vi "calculateWaveformTime.vi"(8 "error in (no error)":errorcluster, 11 "ChirpWave in":refnum<class "ChirpWave.lvclass">) -> (0 "error out":errorcluster, 2 "Waveform Time":dbl[unit], 3 "ChirpWave out":refnum<class "ChirpWave.lvclass">)   [LabVIEW 2015, in "ChirpWave.lvclass"]
uses:
  ChirpWave.lvclass
  ChirpWave.lvclass/ChirpWave.ctl
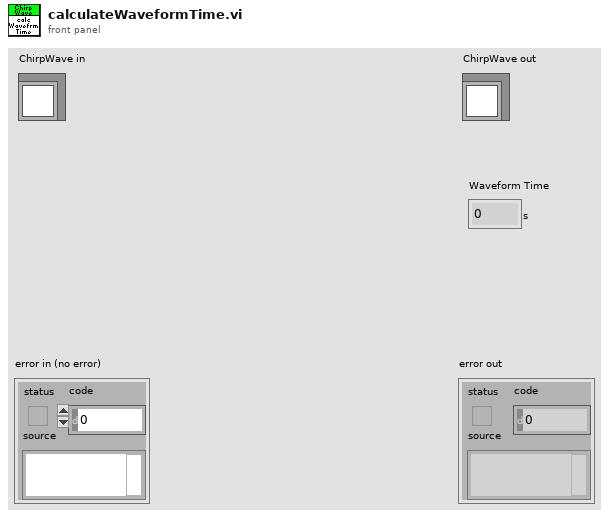
[diagram p1: front panel]
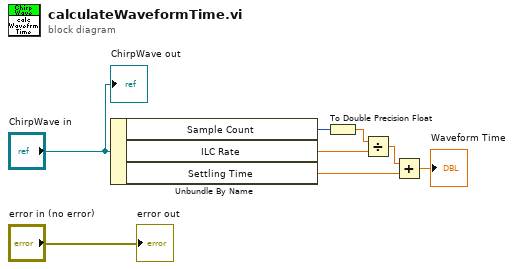
[diagram p0: block diagram]
diagram:
  n1 = Unbundle By Name("ChirpWave in") -> ("Sample Count"=w5:u32, "ILC Rate"=w6:dbl[unit], "Settling Time"=w3:dbl[unit])
  n2 = To Double Precision Float(number=w5) -> (double precision float=w4:dbl)
  n3 = Divide(x=w4, y=w6) -> (x/y=w2:dbl[unit])
  n4 = Add(x=w2, y=w3) -> (x+y=→"Waveform Time":dbl[unit])
  "error out" <- "error in (no error)"
  "ChirpWave out" <- "ChirpWave in"
